vi "Converti_ dati.vi"(11 "String in":string) -> (0 "libero1 2":bool, 1 "libero1":bool, 2 "Check last 2bit(T=OK)":bool, 3 "Converted":dbl, 4 "element":bool, 5 "FS 2":T1={"A"=2.0, "V"=2.0, "TRI\\MONO"=2.0, "A*10?"=FALSE} {"TRI\\MONO" items=["MONOFASE", "TRIFASE"]})   [LabVIEW 2016]
panel:
  out "Boolean array 2":bool[](array[boolean])
  out "Boolean array":bool[](array[boolean])
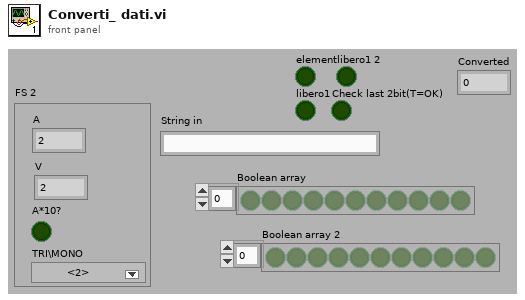
[diagram p1: front panel]
types:
  T1 = cluster{"A":dbl, "V":dbl, "TRI\\MONO":dbl, "A*10?":bool}
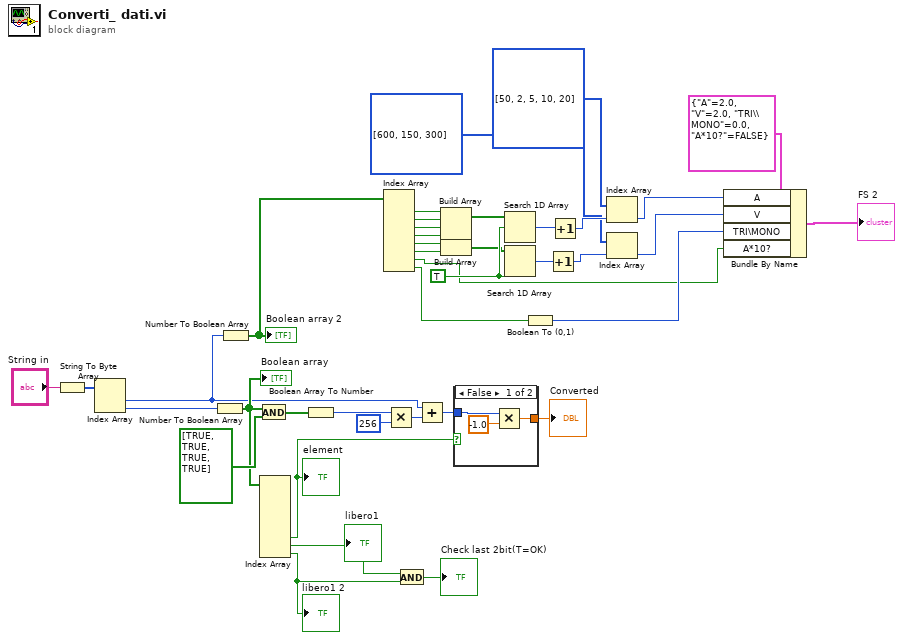
[diagram p0: block diagram]
diagram:
  w19 = TRUE ("element")
  n1 = String To Byte Array(string="String in") -> (unsigned byte array=w38:u8[])
  n2 = Index Array(array=w38) -> (element #1=w24:u8, element #2=w37:u8)  [unwired: 2 in]
  n3 = Number To Boolean Array(number=w37) -> (Boolean array=w31:bool[])
  "Boolean array" <- w31
  n4 = Number To Boolean Array(number=w24) -> (Boolean array=w10:bool[])
  "Boolean array 2" <- w10
  n5 = And(x=w31, y=bool[] [TRUE, TRUE, TRUE, TRUE]) -> (x .and. y?=w35:bool[])
  n6 = Index Array(array=w31) -> (element #6=w30:bool, element #7=w27:bool, element #8=w26:bool)  [unwired: 8 in, 5 out]
  "element" <- w30
  "libero1" <- w27
  "libero1 2" <- w26
  n7 = Boolean Array To Number(Boolean array=w35) -> (number=w34:u32)
  n8 = Index Array(array=w10) -> (element #1=w11:bool, element #2=w12:bool, element #3=w13:bool, element #4=w9:bool, element #5=w14:bool, element #6=w15:bool, element #7=w3:bool, element #8=w5:bool)  [unwired: 8 in]
  n9 = Multiply(x=w34, y=u32 256) -> (x*y=w32:u32)
  n10 = And(x=w27, y=w26) -> (x .and. y?=→"Check last 2bit(T=OK)":bool)
  n11 = Add(x=w24, y=w32) -> (x+y=w29:u32)
  n12 = Build Array(w11, w12, w13, w9) -> (w17:bool[])
  n13 = Build Array(w14, w15) -> (w18:bool[])
  n14 = case shown="False" w30 {
    tunnel: w29 -> [w42 w43]
    tunnel: [w40 w43] -> w28
    frame False {
      n15 = Multiply(x=w42, y=-1.0) -> (x*y=w40:dbl)
    }
    frame True {
    }
  }
  "Converted" <- w28
  n16 = Search 1D Array(1D array=w17, element=w19) -> (index of element=w20:i32)  [unwired: 1 in]
  n17 = Search 1D Array(1D array=w18, element=w19) -> (index of element=w22:i32)  [unwired: 1 in]
  n18 = Boolean To (0,1)(Boolean=w5) -> (0, 1=w4:i16)
  n19 = Increment(x=w22) -> (x+1=w23:i32)
  n20 = Increment(x=w20) -> (x+1=w21:i32)
  n21 = Index Array(array=i32[] [50, 2, 5, 10, 20], index=w21) -> (element=w7:i32)
  n22 = Index Array(array=i32[] [600, 150, 300], index=w23) -> (element=w6:i32)
  n23 = Bundle By Name(cluster=T1 {"A"=2.0, "V"=2.0, "TRI\\MONO"=0.0, "A*10?"=FALSE} ("FS 2"), "A"=w7, "V"=w6, "TRI\\MONO"=w4, "A*10?"=w3) -> (→"FS 2":T1)
